vi "Status.vi"(8 "error in (no error)":errorcluster, 9 "Progress Bar":refnum<vi>, 10 "Status Bar":refnum<vi>, 11 "VI Refnum":refnum<vi>) -> (0 "error out":errorcluster)   [LabVIEW 2019, in "Status.lvlib"]
uses:
  Status.lvlib
  Message Queue/State Name.ctl
  Message Queue/Enqueue (Single).vi
  Message Queue/Reference Queue.vi
  <vilib>/Utility/error.llb/Error Cluster From Error Code.vi
  <vilib>/ErrorRing/Error Ring.xnode
  Message Queue/Message Queue.lvlib
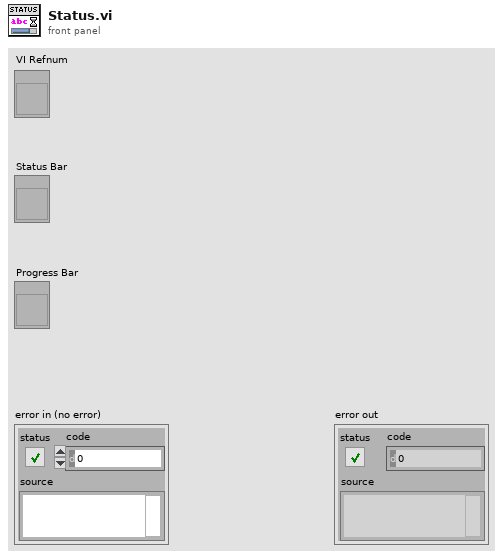
[diagram p1: front panel]
types:
  T1 = typedef "Status.lvlib/State Name.ctl" = enum16{"Initialize", "Update Progress Bar", "Update Status Bar", "Set Cursor Busy", "Unset Cursor Busy", "Error", "Default", "Exit"}
  T2 = typedef "Message Queue.lvlib/State Name.ctl" = enum16{"Default", "Initialize", "Initialize Data", "Initialize Modules", "Initialize Panel", "Close FP", "Open FP", "Initialize Menu", "Mode", "Update Subpanel", "Error", "Open Help", "About", "Open WebResources", "Exit"}
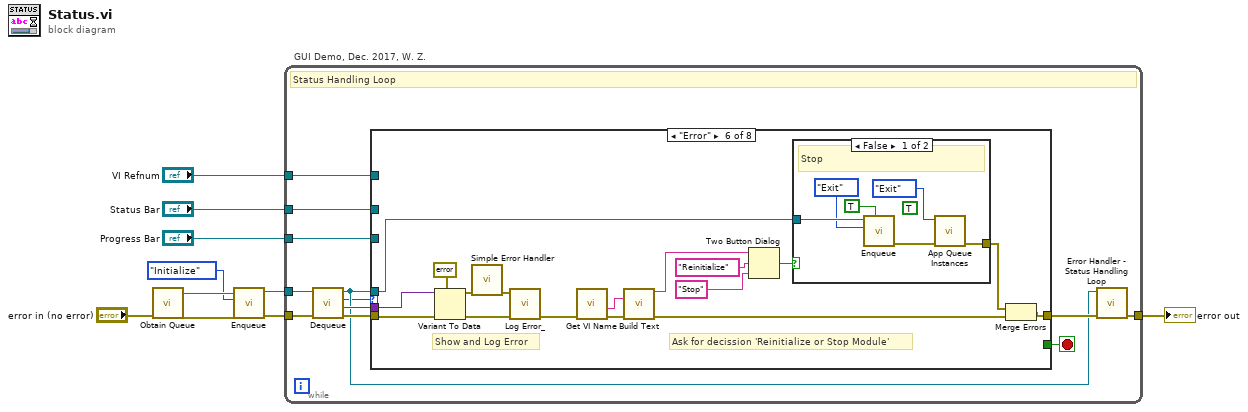
[diagram p0: block diagram]
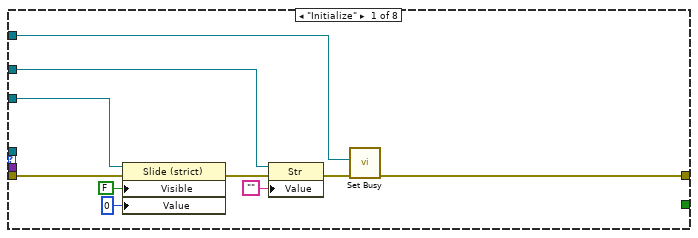
[diagram p2: hidden frame]
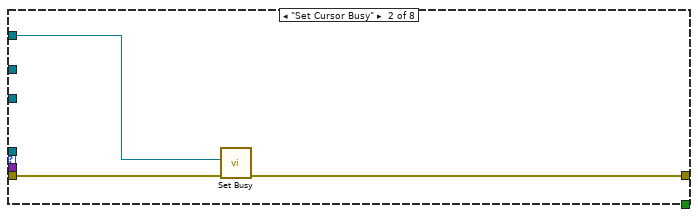
[diagram p3: hidden frame]
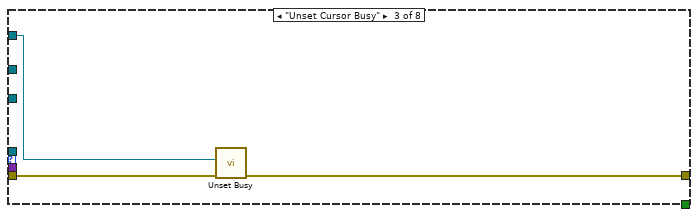
[diagram p4: hidden frame]
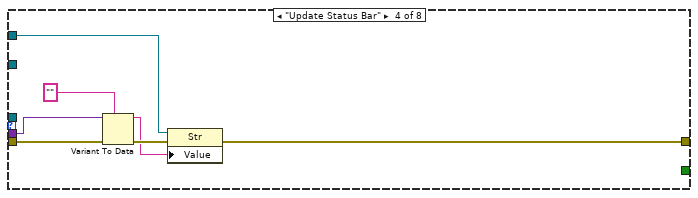
[diagram p5: hidden frame]
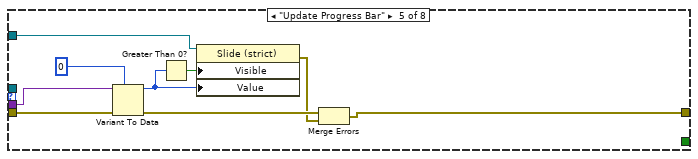
[diagram p6: hidden frame]
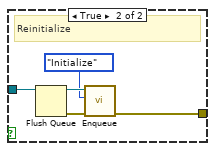
[diagram p7: hidden frame]
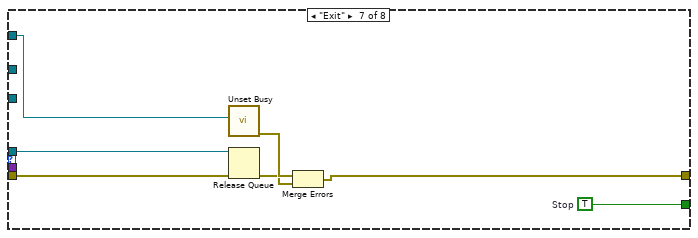
[diagram p8: hidden frame]
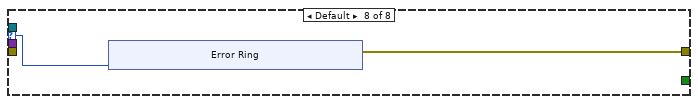
[diagram p9: hidden frame]
diagram:
  # "GUI Demo, Dec. 2017, W. Z."
  n1 = call "Obtain Queue.vi"("error in (no error)"="error in (no error)") -> ("error out"=w10:errorcluster, "queue out"=w9:refnum<queue>)  [unwired: 9 in]
  n2 = call-poly "Enqueue.vi"("error in (no error)"=w10, "States"=State_Name."Initialize", "Message Queue"=w9) -> ("error out"=w8:errorcluster, "dup Message Queue"=w7:refnum<queue>)  [unwired: 7 in]
  n3 = while {
    tunnel: w8 -> [w22]
    tunnel: w7 -> [w21]
    tunnel: [w17] -> w5
    tunnel: "Status Bar" -> [w15]
    tunnel: "VI Refnum" -> [w13]
    tunnel: "Progress Bar" -> [w12]
    stop <- w19 stop-if-true
    # "Status Handling Loop"
    n4 = call "Dequeue.vi"("error in (no error)"=w22, "Message Queue"=w21) -> ("error out"=w20:errorcluster, "Message Data"=w16:variant, "State"=w11:T1, "dup Message Queue"=w14:refnum<queue>)  [unwired: 4 in, 2 out]
    n5 = case shown="\"Error\"" w11 {
      selector: w11 -> [_ _ _ _ _ _ _ w91]
      tunnel: w20 -> [w27 w35 w38 w43 w49 w57 w84 _]
      tunnel: [w25 w34 w37 w45 w47 w58 w86 w90] -> w18
      tunnel: [_ _ _ _ _ _ w89 _] -> w19
      tunnel: w16 -> [_ _ _ w41 w48 w56 _ _]
      tunnel: w15 -> [w29 _ _ w44 _ _ _ _]
      tunnel: w14 -> [_ _ _ _ _ w55 w88 _]
      tunnel: w13 -> [w24 w33 w36 _ _ _ w83 _]
      tunnel: w12 -> [w23 _ _ _ w46 _ _ _]
      frame "Initialize" {
        n6 = property class="Slide (strict)"(reference=w23, error in=w27, "Visible"=FALSE, "Value"=u8 0) -> (error out=w30:errorcluster)  [unwired: 1 out]
        n7 = property class="Str"(reference=w29, error in=w30, "Value"="") -> (error out=w26:errorcluster)  [unwired: 1 out]
        n8 = call <vilib>:"Set Busy.vi"("error in (no error)"=w26, "VI reference (current VI)"=w24) -> ("error out"=w25:errorcluster)  [unwired: 8 in, 1 out]
      }
      frame "Set Cursor Busy" {
        n9 = call <vilib>:"Set Busy.vi"("error in (no error)"=w35, "VI reference (current VI)"=w33) -> ("error out"=w34:errorcluster)  [unwired: 8 in, 1 out]
      }
      frame "Unset Cursor Busy" {
        n10 = call <vilib>:"Unset Busy.vi"("error in (no error)"=w38, "VI reference (current VI)"=w36) -> ("error out"=w37:errorcluster)  [unwired: 9 in]
      }
      frame "Update Status Bar" {
        n11 = Variant To Data(error in=w43, type="", Variant=w41) -> (data=w40:string, error out=w42:errorcluster)
        n12 = property class="Str"(reference=w44, error in=w42, "Value"=w40) -> (error out=w45:errorcluster)  [unwired: 1 out]
      }
      frame "Update Progress Bar" {
        n13 = Variant To Data(error in=w49, type=u8 0 ("Progress Bar"), Variant=w48) -> (data=w52:u8, error out=w51:errorcluster)
        n14 = Greater Than 0?(x=w52) -> (x > 0?=w53:bool)
        n15 = property class="Slide (strict)"(reference=w46, "Visible"=w53, "Value"=w52) -> (error out=w50:errorcluster)  [unwired: 1 in, 1 out]
        n16 = Merge Errors(w51, w50) -> (w47:errorcluster)
      }
      frame "Error" {
        # "Ask for decission 'Reinitialize or Stop Module'"
        # "Show and Log Error"
        n17 = Variant To Data(error in=w57, type=errorcluster {"status"=FALSE, "code"=0, "source"=""} ("error constant"), Variant=w56) -> (data=w62:errorcluster, error out=w69:errorcluster)
        n18 = call <vilib>:"Simple Error Handler.vi"("error in (no error)"=w62) -> ("error out"=w71:errorcluster)  [unwired: 4 in, 4 out]
        n19 = call "Log Error_.vi"("error in"=w69, "Error log to file"=w71) -> ("error out"=w70:errorcluster)  [unwired: 9 in]
        n20 = call "Get VI Name.vi"("error in (no error)"=w70) -> ("error out"=w65:errorcluster, "VI Name without extension"=w66:string)  [unwired: 8 in, 1 out]
        n21 = call "Build Text"("ModuleName"=w66, "error in (no error)"=w65) -> ("Result"=w68:string, "error out"=w67:errorcluster)  [unwired: 12 in]
        n22 = Two Button Dialog(message=w68, 1:"Stop" ("F button name (\"Cancel\")"), 2:"Reinitialize" ("T button name (\"OK\")")) -> (T button?=w64:bool)
        n23 = case shown="False" w64 {
          tunnel: w55 -> [w77 w82]
          tunnel: [w73 w79] -> w63
          frame False {
            (unwired) TRUE ("Priority Message? (F)")
            # "Stop"
            n24 = call-poly "Enqueue.vi"("Priority Message? Array"=TRUE ("Priority Message? (F)"), "States"=State_Name."Exit", "Message Queue"=w77) -> ("error out"=w74:errorcluster)  [unwired: 7 in, 1 out]
            n25 = call-poly "App Queue Instances.vi"("error in (no error)"=w74, "Tasks"=State_Name."Exit") -> ("error out"=w73:errorcluster)  [unwired: 9 in]
          }
          frame True {
            # "Reinitialize"
            n26 = Flush Queue(queue=w82) -> (queue out=w81:refnum<queue>, error out=w80:errorcluster)  [unwired: 1 in, 1 out]
            n27 = call-poly "Enqueue.vi"("error in (no error)"=w80, "States"=State_Name."Initialize", "Message Queue"=w81) -> ("error out"=w79:errorcluster)  [unwired: 7 in, 1 out]
          }
        }
        n28 = Merge Errors(w63, w67) -> (w58:errorcluster)
      }
      frame "Exit" {
        w89 = TRUE  # Stop
        n29 = call <vilib>:"Unset Busy.vi"("VI reference (current VI)"=w83) -> ("error out"=w87:errorcluster)  [unwired: 10 in]
        n30 = Release Queue(queue=w88, error in (no error)=w84) -> (error out=w85:errorcluster)  [unwired: 1 in, 2 out]
        n31 = Merge Errors(w87, w85) -> (w86:errorcluster)
      }
      frame Default {
        n32 = xnode "Error Ring"("parameter 0"=w91) -> ("error out"=w90:errorcluster)
      }
    }
    n33 = call "Error Handler - Status Handling Loop.vi"("error in (no error)"=w18, "Message Queue"=w14) -> ("dup error in"=w17:errorcluster)  [unwired: 8 in, 1 out]
  }
  "error out" <- w5
